vi "Data Replay Simulation Test.vi"() -> ()   [LabVIEW 2013]
uses:
  Data File Loader/AngleReference.ctl
  IP/Analog Data Replay/v1.0.0/Analog Data Replay Load Input.ctl
  <vilib>/rvi/interface/common/niFpgaWaitOnOcc.vi
  <vilib>/rvi/interface/RandomDataEmulation/nirviRandomDataOpen.vi
  <vilib>/rvi/interface/common/niFpgaCacheSessionInfoDynamic.vi
  <vilib>/Utility/error.llb/Error Cluster From Error Code.vi
  <vilib>/rvi/errors/niLvFpgaAdjustHostInterfaceError.vi
  <vilib>/FPGAPlugInAG/Dynamic/niLvFpga_Run_Dynamic.vi
  <vilib>/FPGAPlugInAG/Dynamic/niLvFpga_Close_Dynamic.vi
  <vilib>/rvi/interface/nirviOpenFPGA/nirviOpenFPGA.xnode
  Simulation FPGA/Simulation rate limited APU + 1 Data Replay.vi
  <vilib>/rvi/interface/nirviReadWriteControl/nirviReadWriteControl.xnode
  <vilib>/rvi/interface/nirviMethod/nirviMethod.xnode
  <vilib>/rvi/interface/nirviCloseFPGA/nirviCloseFPGA.xnode
  <userlib>/AES/RT/AES RT.lvlib
  <vilib>/rvi/interface/Simulation/niFpgaSimulationCallBeginRW.vi
  NiFpgaLv.dll
  IP/Analog Data Replay/v1.0.0/Analog Data Replay v1.0.0.lvlib
panel:
  out "Load done":bool
  out "Load time (s)":dbl=9.013101180287777
  in  "RPM Threshold":dbl format="%#_15g"
  in  "Offset":dbl format="%#_15g"
  in  "Reverse Negate":bool
  in  "RPM":dbl=500.0 format="%#_15g"
  in  "stop":bool
  in  "threshold speed (RPM)":dbl
  in  "threshold voltage":dbl=10.0
  in  "maximum speed (RPM)":dbl=10000.0
  in  "maximum voltage":dbl=10.0
  in  "acceleration (RPM/sec)":dbl=inf
  out "Data":dbl[](graph)
  in  "votlage at max RPM":dbl=10.0
  out "Selected Offset":i32=2705
  out "Selected Length":i32=3178
  in  "CycleAngle?":T1
  in  "ReverseData":bool
  in  "MissingTeeth Location":dbl=200.0
  in  "File Path":path=path "C:/Users/sbarrett/Documents/SVN/Engine Simulation/Engine Sim FPGA Example/crank VR data.csv"
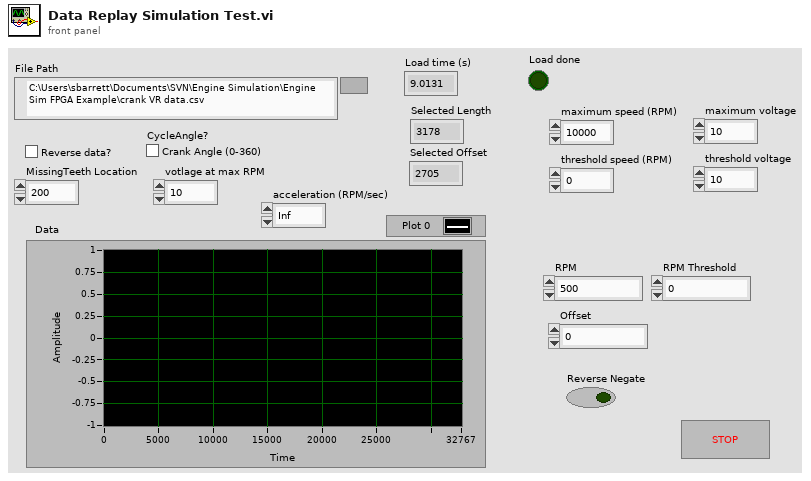
[diagram p1: front panel]
types:
  T1 = typedef "AngleReference.ctl" = bool
  T2 = typedef "Engine Position Simulation.lvlib/Analog Data Replay v1.0.0.lvlib/Analog Data Replay Load Input.ctl" = cluster{"Data":i16[], "LoadOffset":u16, "Done":bool}
  T3 = cluster{"maximum cycle angle (degrees)":fxp<+,18,11>}
  T4 = cluster{"ReverseNegate":bool, "CycleAngle":bool, "AngleToAddress":fxp<+,18,7>, "RPMThreshold":fxp<+/-,22,-6>, "ThresholdValue":i16}
  T5 = cluster{"acceleration (degrees/tic^2)":fxp<+,19,-28>, "crank start angle (degrees)":fxp<+,16,9>, "cycle start angle (degrees)":fxp<+,18,11>}
  T6 = cluster{"desired speed (degrees/tic)":fxp<+/-,22,-6>, "reset":bool}
  T7 = cluster{"Offset":fxp<+,18,11>, "VScaleSlope":fxp<+,18,12>, "VScaleIntercept":fxp<+/-,18,3>}
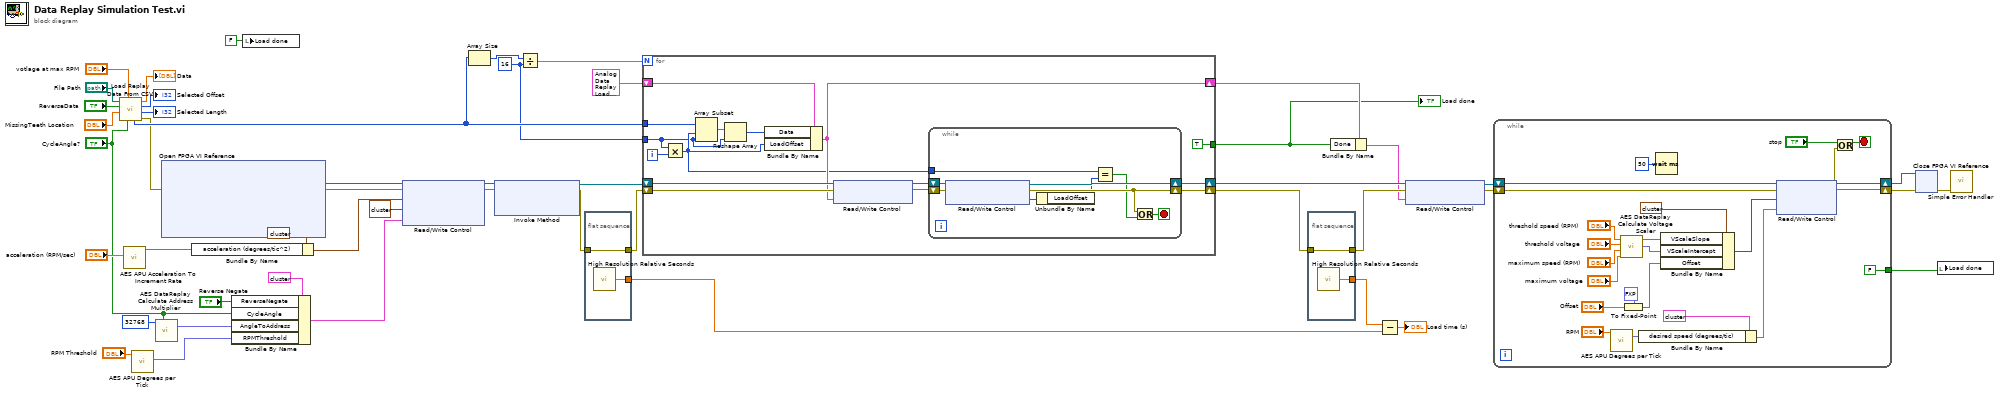
[diagram p0: block diagram]
diagram:
  w8 = 16 ("y")
  n1 = call "Load Replay Data From CSV.vi"("CycleAngle?"="CycleAngle?", "votlage at max RPM"="votlage at max RPM", "MissingTeeth Location"="MissingTeeth Location", "ReverseData"="ReverseData", "File Path"="File Path") -> ("error out"=w25:errorcluster, "Selected Length"=→"Selected Length":i32, "Selected Offset"=→"Selected Offset":i32, "Data"=→"Data":dbl[], "DAC data"=w49:i16[])  [unwired: 2 in]
  n2 = call <userlib>:"AES APU Acceleration To Increment Rate.vi"("acceleration (RPM/sec)"="acceleration (RPM/sec)") -> ("increment rate"=w32:fxp<+/-,47,-4>)  [unwired: 10 in]
  n3 = call <userlib>:"AES APU Degrees per Tick.vi"("RPM"="RPM Threshold") -> ("degrees per tick"=w26:fxp<+/-,47,-4>)  [unwired: 9 in, 1 out]
  n4 = call <userlib>:"AES DataReplay Calculate Address Multiplier.vi"("CycleAngle?"="CycleAngle?", "memory size (divisible by 32)"=32768) -> ("angle to address multiplier"=w29:fxp<+,18,7>)  [unwired: 9 in]
  n5 = xnode "Open FPGA VI Reference"("error in"=w25) -> ("FPGA VI Reference Out"=w4:refnum<k20>, "error out"=w45:errorcluster)  [unwired: 1 in]
  n6 = Bundle By Name(cluster=T5 {"acceleration (degrees/tic^2)"=0.0, "crank start angle (degrees)"=0.0, "cycle start angle (degrees)"=0.0} ("my apu"), "acceleration (degrees/tic^2)"=w32) -> (w44:T5)
  n7 = Bundle By Name(cluster=T4 {"ReverseNegate"=FALSE, "CycleAngle"=FALSE, "AngleToAddress"=0.0, "RPMThreshold"=0.0, "ThresholdValue"=0} ("my replay"), "ReverseNegate"="Reverse Negate", "CycleAngle"="CycleAngle?", "AngleToAddress"=w29, "RPMThreshold"=w26) -> (w43:T4)
  n8 = local write "Load done"(FALSE ("Load done")) -> ()
  n9 = xnode "Read/Write Control"("FPGA VI Reference In"=w4, "error in"=w45, "my apu settings"=w44, "global settings"=T3 {"maximum cycle angle (degrees)"=720.0}, "my replay settings"=w43) -> ("FPGA VI Reference Out"=w20:refnum<k20>, "error out"=w2:errorcluster)
  n10 = Array Size(array=w49) -> (size(s)=w21:i32)
  n11 = xnode "Invoke Method"("FPGA VI Reference In"=w20, "error in"=w2) -> ("FPGA VI Reference Out"=w19:refnum<k20>, "error out"=w17:errorcluster)  [unwired: 1 in]
  n12 = Divide(x=w21, y=w8) -> (x/y=w22:dbl)
  n13 = flat-sequence {
    tunnel: [w51] -> w18
    tunnel: w17 -> [w51]
    tunnel: [w50] -> w13
    frame #0 {
      n14 = call <vilib>:"High Resolution Relative Seconds.vi"() -> ("relative seconds"=w50:dbl)
    }
  }
  n15 = for {
    N: w22 -> [_]
    shift-right: [w56] -> w16
    shift-left: w18 -> [w63]
    tunnel: w49 -> [w66]
    tunnel: w8 -> [w52]
    shift-right: [w57] -> w10
    shift-left: w19 -> [w62]
    shift-right: [w54] -> w7
    shift-left: T2 {"Data"=[0, 0, 0, 0, 0, 0, 0, 0, 0, 0, 0, 0, 0, 0, 0, 0], "LoadOffset"=0, "Done"=FALSE} ("analog data replay load input v1.0.0") -> [w59]
    tunnel: [TRUE ("Done")] -> w3
    i -> [w64]
    n16 = Multiply(x=w52, y=w64) -> (x*y=w53:i32)
    n17 = Array Subset(array=w66, index=w53, length=w52) -> (w65:i16[])
    n18 = Reshape Array(w65, w52) -> (w58:i16[])
    n19 = Bundle By Name(cluster=w59, "Data"=w58, "LoadOffset"=w53) -> (w54:T2)
    n20 = xnode "Read/Write Control"("FPGA VI Reference In"=w62, "error in"=w63, "my replay load in"=w54) -> ("FPGA VI Reference Out"=w61:refnum<k20>, "error out"=w60:errorcluster)
    n21 = while {
      shift-right: [w71] -> w56
      shift-left: w60 -> [w75]
      shift-right: [w73] -> w57
      shift-left: w61 -> [w74]
      tunnel: w53 -> [w67]
      stop <- w72 stop-if-true
      n22 = xnode "Read/Write Control"("FPGA VI Reference In"=w74, "error in"=w75) -> ("FPGA VI Reference Out"=w73:refnum<k20>, "error out"=w71:errorcluster, "my replay load out"=w70:cluster{"LoadOffset":u16})
      n23 = Unbundle By Name(w70) -> ("LoadOffset"=w69:u16)
      n24 = Equal?(x=w67, y=w69) -> (x = y?=w68:bool)
      n25 = Or(x=w71, y=w68) -> (x .or. y?=w72:bool)
    }
  }
  "Load done" <- w3
  n26 = flat-sequence {
    tunnel: [w77] -> w15
    tunnel: w16 -> [w77]
    tunnel: [w76] -> w14
    frame #0 {
      n27 = call <vilib>:"High Resolution Relative Seconds.vi"() -> ("relative seconds"=w76:dbl)
    }
  }
  n28 = Bundle By Name(cluster=w7, "Done"=w3) -> (w6:T2)
  n29 = Subtract(x=w14, y=w13) -> (x-y=→"Load time (s)":dbl)
  n30 = xnode "Read/Write Control"("FPGA VI Reference In"=w10, "error in"=w15, "my replay load in"=w6) -> ("FPGA VI Reference Out"=w9:refnum<k20>, "error out"=w11:errorcluster)
  n31 = while {
    shift-right: [w88] -> w48
    shift-left: w11 -> [w100]
    shift-right: [w94] -> w47
    shift-left: w9 -> [w99]
    tunnel: [FALSE ("Load")] -> w24
    stop <- w89 stop-if-true
    n32 = call <userlib>:"AES APU Degrees per Tick.vi"("RPM"="RPM") -> ("degrees per tick"=w80:fxp<+/-,47,-4>)  [unwired: 9 in, 1 out]
    n33 = call <userlib>:"AES DataReplay Calculate Voltage Scaler.vi"("maximum voltage"="maximum voltage", "maximum speed (RPM)"="maximum speed (RPM)", "threshold voltage"="threshold voltage", "threshold speed (RPM)"="threshold speed (RPM)") -> ("intercept (b)"=w84:fxp<+/-,18,3>, "slope (m)"=w85:fxp<+,18,12>)  [unwired: 6 in]
    n34 = To Fixed-Point(fixed-point type=fxp<+/-,61,10> 0.0 ("FullyCustomTeeth.Cams.Cam1.Offset"), number="Offset") -> (fixed-point=w83:fxp<+/-,61,10>)
    n35 = Bundle By Name(cluster=T6 {"desired speed (degrees/tic)"=0.0, "reset"=FALSE} ("my apu"), "desired speed (degrees/tic)"=w80) -> (w79:T6)
    n36 = Wait (ms)(milliseconds to wait=u32 50) -> ()  [unwired: 1 out]
    n37 = Bundle By Name(cluster=T7 {"Offset"=0.0, "VScaleSlope"=0.0, "VScaleIntercept"=0.0} ("my replay"), "VScaleSlope"=w85, "VScaleIntercept"=w84, "Offset"=w83) -> (w82:T7)
    n38 = xnode "Read/Write Control"("FPGA VI Reference In"=w99, "error in"=w100, "my replay in"=w82, "my apu in"=w79) -> ("FPGA VI Reference Out"=w94:refnum<k20>, "error out"=w88:errorcluster)
    n39 = Or(x="stop", y=w88) -> (x .or. y?=w89:bool)
  }
  n40 = xnode "Close FPGA VI Reference"("FPGA VI Reference In"=w47, "error in"=w48) -> ("error out"=w46:errorcluster)
  n41 = local write "Load done"(w24) -> ()
  n42 = call <vilib>:"Simple Error Handler.vi"("error in (no error)"=w46) -> ()  [unwired: 4 in, 5 out]
